vi "subFilterForExporters.vi"(8 "error in (no error)":errorcluster, 9 "Addons":path[](array[path]), 11 "UIManager in":refnum<class "UIManager.lvclass">) -> (0 "error out":errorcluster, 3 "UIManager out":refnum<class "UIManager.lvclass">)   [LabVIEW 2020, in "UserInterface.lvlib" / "UIManager.lvclass"]
uses:
  UIManager.lvclass
  UIManager.lvclass/UIManager.ctl
  <vilib>/Utility/LVClass/Get LV Class Default Value.vi
  ExtensionInterfaces/IExporter/IExporter.lvclass
  e42b8347-b43a-46fd-a3a0-476dc182b4c2.vi
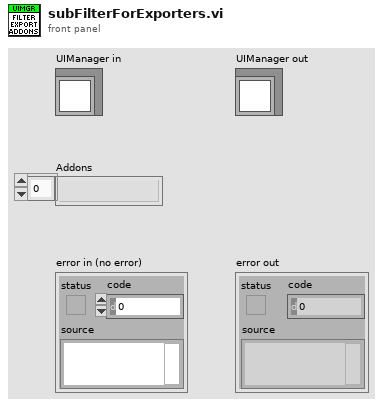
[diagram p1: front panel]
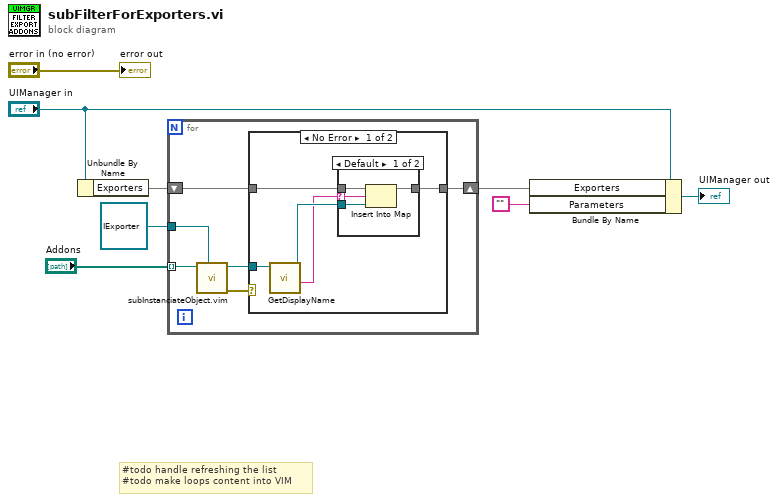
[diagram p0: block diagram]
diagram:
  # "#todo handle refreshing the list\n#todo make loops content into VIM"
  n1 = Unbundle By Name("UIManager in") -> ("Exporters"=w4:map{string, refnum<class "IExporter.lvclass">})
  n2 = for {
    tunnel: "Addons" -> [w12] mode=indexing
    shift-right: [w13] -> w1
    shift-left: w4 -> [w14]
    tunnel: refnum<class "IExporter.lvclass"> refnum ("ExtensionInterfaces.lvlib:IExporter.lvclass") -> [w11]
    n3 = call "subInstanciateObject.vim"("Target object"=w11, "Class path"=w12) -> ("error out"=w9:errorcluster, "Object"=w10:refnum<class "IExporter.lvclass">)  [unwired: 8 in]
    n4 = case shown="No Error" w9 {
      tunnel: w14 -> [w18 w25]
      tunnel: w10 -> [w19 _]
      tunnel: [w16 w25] -> w13
      frame No Error {
        n5 = call-dynamic "GetDisplayName.vi"("IExporter in"=w19) -> ("Display name"=w15:string, "IExporter out"=w17:refnum<class "IExporter.lvclass">)  [unwired: 8 in, 1 out]
        n6 = case shown="Default" w15 {
          selector: w15 -> [w20 _]
          tunnel: w18 -> [w23 w24]
          tunnel: w17 -> [w22 _]
          tunnel: [w21 w24] -> w16
          frame Default {
            n7 = Insert Into Map(map in=w23, key=w20, value=w22) -> (map out=w21:map{string, refnum<class "IExporter.lvclass">})  [unwired: 2 out]
          }
          frame "" {
          }
        }
      }
      frame Error {
      }
    }
  }
  n8 = Bundle By Name(cluster="UIManager in", "Exporters"=w1, "Parameters"="") -> (→"UIManager out":refnum<class "UIManager.lvclass">)
  "error out" <- "error in (no error)"
